vi "openMethodViReference.vi"(8 "error in (no error)":errorcluster, 11 "TestCase in":refnum<class "TestCase.lvclass">) -> (0 "error out":errorcluster, 3 "TestCase out":refnum<class "TestCase.lvclass">)   [LabVIEW 2013, in "TestCase.lvclass"]
uses:
  TestCase.lvclass
  TestCase.lvclass/TestCase.ctl
  private/testMethodName.ctl
  JKI Reuse/Filter Error Codes (Scalar)__jki_lib_error_handling -- VI Tester.vi
  Libraries/VITesterUtilities.lvlib
panel:
  # "JKI VI Tester for LabVIEW\nhttp://jkisoft.com/vi-tester\nCopyright (C) 2007-2009, JKI <info@jkisoft.com>\nALL RIGHTS RESERVED"
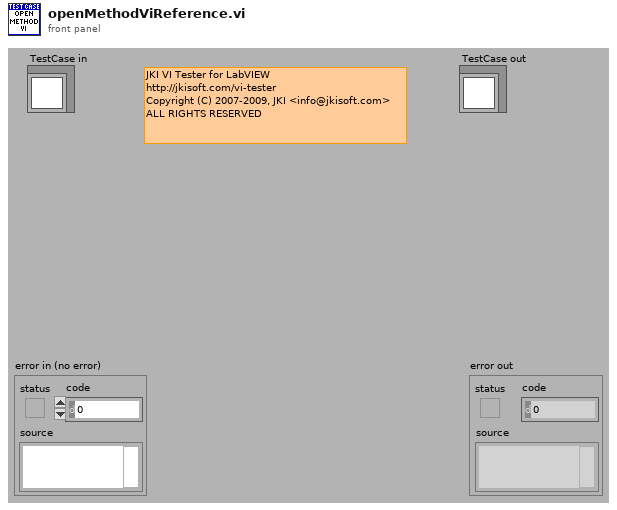
[diagram p1: front panel]
types:
  T1 = typedef "TestCase.lvclass/testMethodName.ctl" = string
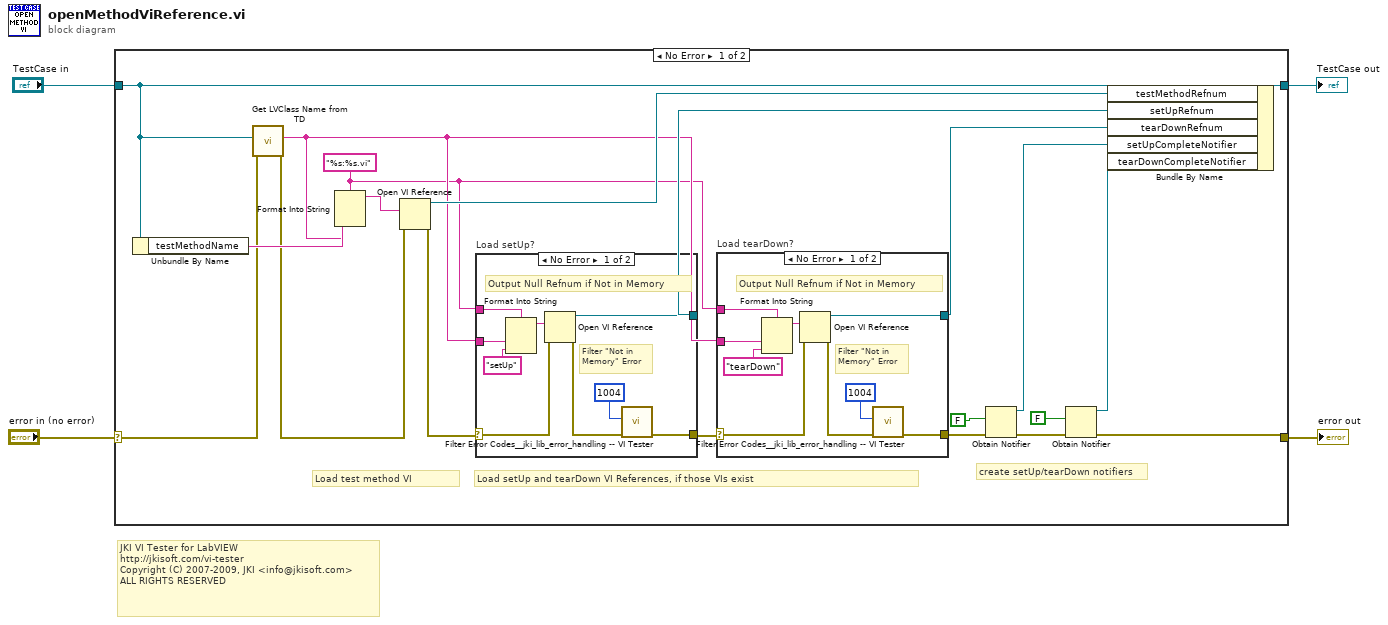
[diagram p0: block diagram]
diagram:
  # "JKI VI Tester for LabVIEW\nhttp://jkisoft.com/vi-tester\nCopyright (C) 2007-2009, JKI <info@jkisoft.com>\nALL RIGHTS RESERVED"
  n1 = case shown="No Error" "error in (no error)" {
    selector: "error in (no error)" -> [w18 w46]
    tunnel: [w8 w46] -> w3
    tunnel: [w20 w45] -> w1
    tunnel: "TestCase in" -> [w19 w45]
    frame No Error {
      w12 = "%s:%s.vi" ("format string")
      # "create setUp/tearDown notifiers"
      # "Load test method VI"
      # "Load setUp and tearDown VI References, if those VIs exist"
      n2 = Unbundle By Name(w19) -> ("testMethodName"=w24:T1)
      n3 = call "Get LVClass Name from TD.vi"("error in"=w18, "Variant"=w19) -> ("error out"=w22:errorcluster, "LVClass Name"=w13:string)  [unwired: 8 in]
      n4 = Format Into String(format string=w12, w13, w24) -> (resulting string=w23:string)  [unwired: 2 in, 1 out]
      n5 = Open VI Reference(vi path=w23, error in (no error)=w22) -> (vi reference=w21:refnum<vi>, error out=w16:errorcluster)  [unwired: 4 in]
      n6 = case "Load setUp?" shown="No Error" w16 {
        selector: w16 -> [w38 w44]
        tunnel: [w41 _] -> w17
        tunnel: w12 -> [w40 _]
        tunnel: [w36 w44] -> w15
        tunnel: w13 -> [w39 _]
        frame No Error {
          # "Output Null Refnum if Not in Memory"
          # "Filter \"Not in Memory\" Error"
          n7 = Format Into String(format string=w40, w39, T1 "setUp" ("input 2")) -> (resulting string=w42:string)  [unwired: 2 in, 1 out]
          n8 = Open VI Reference(vi path=w42, error in (no error)=w38) -> (vi reference=w41:refnum<vi>, error out=w37:errorcluster)  [unwired: 4 in]
          n9 = call-poly "Filter Error Codes__jki_lib_error_handling -- VI Tester.vi"("error in"=w37, "error code to filter"=1004) -> ("error out"=w36:errorcluster)  [unwired: 7 in, 2 out]
        }
        frame Error {
        }
      }
      n10 = case "Load tearDown?" shown="No Error" w15 {
        selector: w15 -> [w28 w34]
        tunnel: [w31 _] -> w14
        tunnel: w12 -> [w30 _]
        tunnel: [w26 w34] -> w7
        tunnel: w13 -> [w29 _]
        frame No Error {
          # "Output Null Refnum if Not in Memory"
          # "Filter \"Not in Memory\" Error"
          n11 = Format Into String(format string=w30, w29, T1 "tearDown" ("input 2")) -> (resulting string=w32:string)  [unwired: 2 in, 1 out]
          n12 = Open VI Reference(vi path=w32, error in (no error)=w28) -> (vi reference=w31:refnum<vi>, error out=w27:errorcluster)  [unwired: 4 in]
          n13 = call-poly "Filter Error Codes__jki_lib_error_handling -- VI Tester.vi"("error in"=w27, "error code to filter"=1004) -> ("error out"=w26:errorcluster)  [unwired: 7 in, 2 out]
        }
        frame Error {
        }
      }
      n14 = Obtain Notifier(notification data type=FALSE, error in (no error)=w7) -> (notifier out=w6:refnum<notifier>, error out=w9:errorcluster)  [unwired: 2 in, 1 out]
      n15 = Obtain Notifier(notification data type=FALSE, error in (no error)=w9) -> (notifier out=w5:refnum<notifier>, error out=w8:errorcluster)  [unwired: 2 in, 1 out]
      n16 = Bundle By Name(cluster=w19, "testMethodRefnum"=w21, "setUpRefnum"=w17, "tearDownRefnum"=w14, "setUpCompleteNotifier"=w6, "tearDownCompleteNotifier"=w5) -> (w20:refnum<class "TestCase.lvclass">)
    }
    frame Error {
    }
  }
  "error out" <- w3
  "TestCase out" <- w1
